vi "State Determination.vi"(9 "Time Done":bool, 10 "Current State":T1, 11 "Queue in":refnum<queue>) -> (3 "Queue out":refnum<queue>)   [LabVIEW 2012]
uses:
  Controls/Traffic Light States (with Walk and Exit State).ctl
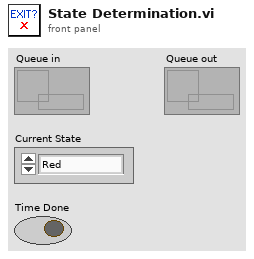
[diagram p1: front panel]
types:
  T1 = typedef "Traffic Light States (with Walk and Exit State).ctl" = enum16{"Red", "RedAmber", "Green", "Amber", "Walk", "Exit"}
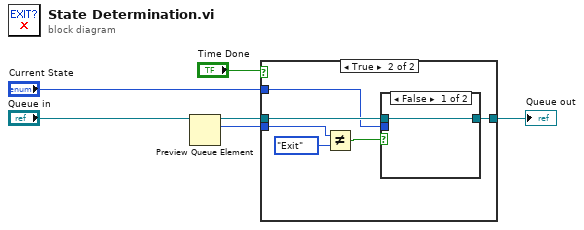
[diagram p0: block diagram]
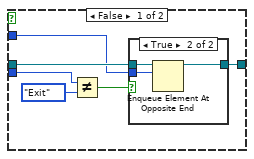
[diagram p2: hidden frame]
diagram:
  n1 = Preview Queue Element(queue="Queue in") -> (queue out=w3:refnum<queue>, element=w4:T1)  [unwired: 2 in, 2 out]
  n2 = case shown="True" "Time Done" {
    tunnel: w3 -> [w9 w19]
    tunnel: w4 -> [w11 w21]
    tunnel: "Current State" -> [w8 w17]
    tunnel: [w7 w18] -> w6
    frame False {
      n3 = Not Equal?(x=w11, y=Traffic_Light_States_(with_Walk_and_Exit_State)."Exit" ("Traffic Light States")) -> (x != y?=w10:bool)
      n4 = case shown="True" w10 {
        tunnel: w9 -> [w13 w16]
        tunnel: w8 -> [_ w15]
        tunnel: [w13 w14] -> w7
        frame False {
        }
        frame True {
          n5 = Enqueue Element At Opposite End(queue=w16, element=w15) -> (queue out=w14:refnum<queue>)  [unwired: 2 in, 2 out]
        }
      }
    }
    frame True {
      n6 = Not Equal?(x=w21, y=Traffic_Light_States_(with_Walk_and_Exit_State)."Exit" ("Traffic Light States")) -> (x != y?=w20:bool)
      n7 = case shown="False" w20 {
        tunnel: w19 -> [w23 w24]
        tunnel: [w23 w24] -> w18
        tunnel: w17 -> [_ _]
        frame False {
        }
        frame True {
        }
      }
    }
  }
  "Queue out" <- w6
